vi "dvp Vi Get Exposure.vi"(10 "pExposure":dbl, 11 "handle":u32) -> (2 "pExposure out":dbl, 3 "function return":u32(ring))   [LabVIEW 2018, in "LabViewDVPCamera.lvlib"]
doc: "LabviewDvp2Api dvpStatus dvpViGetExposure(dvpHandle handle, double *pExposure);"
uses:
  LabViewDVPCamera.lvlib
  LabViewDVPCamera/LabViewDVPCamera.dll
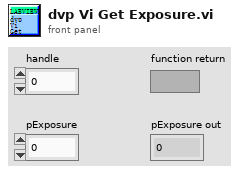
[diagram p1: front panel]
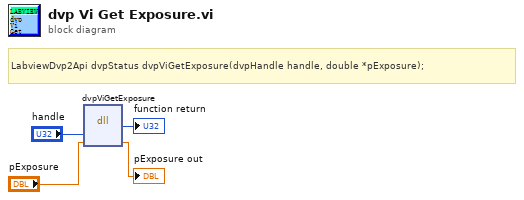
[diagram p0: block diagram]
diagram:
  # "LabviewDvp2Api dvpStatus dvpViGetExposure(dvpHandle handle, double *pExposure);"
  n1 = dll-call lib="C:/Program Files (x86)/DVP2 Labview cn 64/Sample/LabViewDVPCamera/LabViewDVPCamera.*" fn="dvpViGetExposure"("handle"="handle", "pExposure"="pExposure") -> (→"function return":u32, "pExposure"=→"pExposure out":dbl)  [unwired: 4 in, 2 out]
